vi "Get Engine Ref.vi"(8 "error in (no error)":errorcluster, 11 "TSEngine in":refnum<class "Engine.lvclass">) -> (0 "error out":errorcluster, 2 "Engine":refnum<k7>, 3 "TSEngine out":refnum<class "Engine.lvclass">)   [LabVIEW 2020, in "TSS.lvlib" / "Engine.lvclass"]
uses:
  Engine.lvclass
  Engine.lvclass/Engine.ctl
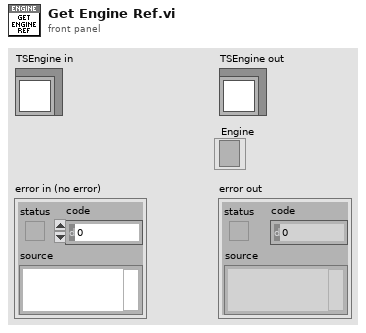
[diagram p1: front panel]
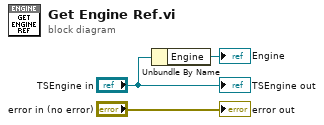
[diagram p0: block diagram]
diagram:
  n1 = Unbundle By Name("TSEngine in") -> ("Engine"=→"Engine":refnum<k7>)
  "error out" <- "error in (no error)"
  "TSEngine out" <- "TSEngine in"
